vi "CopyImageNoMaskGreyscale.vi"(8 "error in (no error)":errorcluster, 10 "Greyscale Image Destination":refnum<data-value>, 11 "Greyscale Image Source":refnum<data-value>) -> (0 "error out":errorcluster, 3 "Greyscale Image Destination (duplicate)":refnum<data-value>)   [LabVIEW 2020, in "g_ar_toolkit.image.lvlib"]
uses:
  g_ar_toolkit.image.lvlib
  c92252ab-1097-45af-a449-7a3c8cf05290.vi
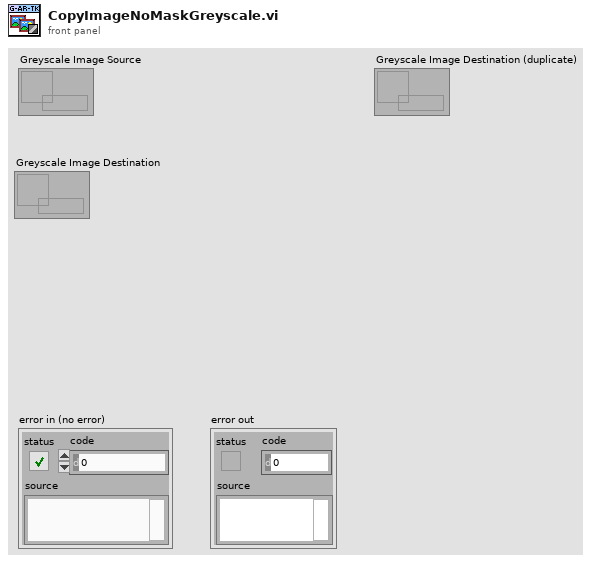
[diagram p1: front panel]
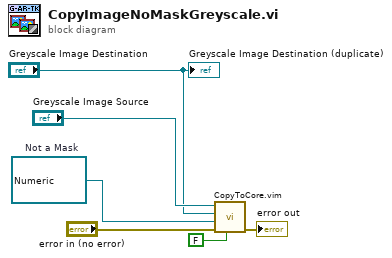
[diagram p0: block diagram]
diagram:
  w1 = refnum<data-value> refnum  # Not a Mask
  n1 = call "CopyToCore.vim"("Has Mask"=FALSE, "error in (no error)"="error in (no error)", "Mask"=w1, "Dst"="Greyscale Image Destination", "Src"="Greyscale Image Source") -> ("error out"=→"error out":errorcluster)  [unwired: 6 in]
  "Greyscale Image Destination (duplicate)" <- "Greyscale Image Destination"
